vi "Calibration.vi"() -> ()   [LabVIEW 2013]
uses:
  <vilib>/Rock Robotics/WPI/Joystick/WPI_JoystickGetSetRefNum.vi
  Globals/Useful Values.vi
  Globals/Homes.vi
  <vilib>/Utility/file.llb/Write To Spreadsheet File (DBL).vi
panel:
  out "Winch Home":dbl=0.95
  out "Intake Home":dbl=0.1
  out "Arm Home":dbl=0.4
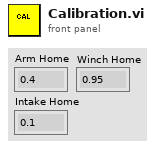
[diagram p1: front panel]
types:
  T1 = typedef "WPI_AnalogChannelDevRef.ctl" = cluster{"DevStatus":errorcluster, "Analog Module":T2, "Analog Channel":T3}
  T2 = typedef "FPGA_TypedefAnalogModule.ctl" = enum16{"Analog Module 1", "Analog Module 2"}
  T3 = typedef "FPGA_AIChannel.ctl" = enum8{"AI 1", "AI 2", "AI 3", "AI 4", "AI 5", "AI 6", "AI 7", "AI 8", "Invalid"}
  T4 = typedef "WPI_JoystickDevRef.ctl" = cluster{"Device":T5}
  T5 = typedef "WPI_JoystickDeviceEnum.ctl" = enum16{"USB 1", "USB 2", "USB 3", "USB 4", "Kinect 1", "Kinect 2"}
  T6 = typedef "WPI_MotorControlDeviceRef.ctl" = cluster{"DeviceStatus":errorcluster, "Type":enum16{"PWM", "CAN"}, "PWM":cluster{"Digital Module":T7, "PWM Channel":T8, "DeadBand":T9}, "CAN":cluster{"Device Number":u8, "Control Mode":T10, "Semaphore":T11, "Max Vout":dbl}, "Invert":bool, "TransformRef":T12, "InvTransformRef":T12}
  T7 = typedef "FPGA_TypedefDigitalModule.ctl" = enum16{"Digital Module 1", "Digital Module 2"}
  T8 = typedef "FPGA_DIOPWMChannel.ctl" = enum8{"PWM 1", "PWM 2", "PWM 3", "PWM 4", "PWM 5", "PWM 6", "PWM 7", "PWM 8", "PWM 9", "PWM 10", "Invalid"}
  T9 = typedef "WPI_PWMDeadband.ctl" = cluster{"Name":string, "maxPositivePwm":i32, "minPositivePwm":i32, "centerPwm":i32, "maxNegativePwm":i32, "minNegativePwm":i32, "angularRange":u16}
  T10 = typedef "WPI_CANJaguar_ControlMode.ctl" = enum8{"Percent VBus", "Current", "Speed", "Position", "Voltage"}
  T11 = typedef "Semaphore RefNum" = refnum<k1>
  T12 = typedef "WPI_PWMTransform_ConPane.ctl" = refnum<vi>
  T13 = typedef "WPI_JoystickButtonState.ctl" = cluster{"Button 1":bool, "Button 2":bool, "Button 3":bool, "Button 4":bool, "Button 5":bool, "Button 6":bool, "Button 7":bool, "Button 8":bool, "Button 9":bool, "Button 10":bool, "Button 11":bool, "Button 12":bool}
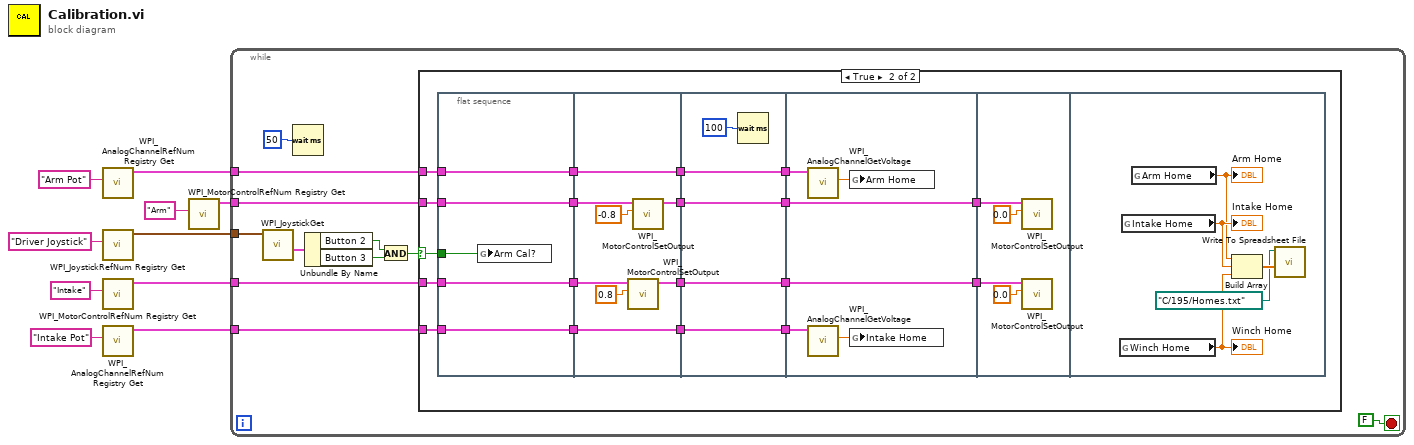
[diagram p0: block diagram]
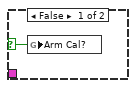
[diagram p2: hidden frame]
diagram:
  n1 = call <vilib>:"WPI_AnalogChannelRefNum Registry Get.vi"("refnum name"="Arm Pot") -> ("AIDeviceRef"=w7:T1)  [unwired: 9 in, 1 out]
  n2 = call <vilib>:"WPI_JoystickRefNum Registry Get.vi"("refnum name"="Driver Joystick") -> ("JoystickDevRef"=w10:T4)  [unwired: 9 in, 1 out]
  n3 = call <vilib>:"WPI_MotorControlRefNum Registry Get.vi"("refnum name"="Intake") -> ("MotorControlDevRef"=w2:T6)  [unwired: 9 in, 1 out]
  n4 = call <vilib>:"WPI_AnalogChannelRefNum Registry Get.vi"("refnum name"="Intake Pot") -> ("AIDeviceRef"=w1:T1)  [unwired: 9 in, 1 out]
  n5 = call <vilib>:"WPI_MotorControlRefNum Registry Get.vi"("refnum name"="Arm") -> ("MotorControlDevRef"=w5:T6)  [unwired: 9 in, 1 out]
  n6 = while {
    tunnel: w10 -> [w20]
    tunnel: w7 -> [w16]
    tunnel: w5 -> [w15]
    tunnel: w2 -> [w12]
    tunnel: w1 -> [w11]
    stop <- FALSE stop-if-true
    n7 = call <vilib>:"WPI_JoystickGet.vi"("JoystickDevRef"=w20) -> ("Buttons"=w19:T13)  [unwired: 4 in, 2 out]
    n8 = Wait (ms)(milliseconds to wait=u32 50) -> ()  [unwired: 1 out]
    n9 = Unbundle By Name(w19) -> ("Button 2"=w18:bool, "Button 3"=w17:bool)
    n10 = And(x=w18, y=w17) -> (x .and. y?=w14:bool)
    n11 = case shown="True" w14 {
      selector: w14 -> [w22 w41]
      tunnel: w16 -> [_ w40]
      tunnel: w15 -> [_ w39]
      tunnel: w12 -> [_ w30]
      tunnel: w11 -> [_ w26]
      frame False {
        n12 = global write "Useful Values.vi" "Arm Cal?"(w22) -> ()
      }
      frame True {
        n13 = flat-sequence {
          tunnel: w41 -> [w46]
          tunnel: [w45] -> w38
          tunnel: w40 -> [w45]
          tunnel: w39 -> [w44]
          tunnel: [w44] -> w37
          tunnel: [w43] -> w31
          tunnel: w30 -> [w43]
          tunnel: [w42] -> w27
          tunnel: w26 -> [w42]
          tunnel: w38 -> [w54]
          tunnel: [w54] -> w35
          tunnel: w37 -> [w52]
          tunnel: [w51] -> w33
          tunnel: w31 -> [w50]
          tunnel: [w48] -> w28
          tunnel: w27 -> [w48]
          tunnel: [w47] -> w25
          tunnel: w35 -> [w59]
          tunnel: [w59] -> w34
          tunnel: w33 -> [w58]
          tunnel: [w58] -> w32
          tunnel: [w56] -> w29
          tunnel: w28 -> [w56]
          tunnel: w25 -> [w55]
          tunnel: [w55] -> w24
          tunnel: w34 -> [w63]
          tunnel: [w65] -> w36
          tunnel: w32 -> [w65]
          tunnel: w29 -> [w62]
          tunnel: w24 -> [w60]
          tunnel: [w60] -> w23
          tunnel: w36 -> [w68]
          tunnel: w23 -> [w66]
          frame #0 {
            n14 = global write "Useful Values.vi" "Arm Cal?"(w46) -> ()
          }
          frame #1 {
            n15 = call <vilib>:"WPI_MotorControlSetOutput.vi"("Output"=0.8, "MotorControlDevRef"=w50) -> ("MotorControlDevRef"=w47:T6)  [unwired: 7 in, 2 out]
            n16 = call <vilib>:"WPI_MotorControlSetOutput.vi"("Output"=-0.8, "MotorControlDevRef"=w52) -> ("MotorControlDevRef"=w51:T6)  [unwired: 7 in, 2 out]
          }
          frame #2 {
            n17 = Wait (ms)(milliseconds to wait=u32 100) -> ()  [unwired: 1 out]
          }
          frame #3 {
            n18 = call <vilib>:"WPI_AnalogChannelGetVoltage.vi"("AIDeviceRef"=w63) -> ("Voltage"=w64:dbl)  [unwired: 8 in, 2 out]
            n19 = call <vilib>:"WPI_AnalogChannelGetVoltage.vi"("AIDeviceRef"=w62) -> ("Voltage"=w61:dbl)  [unwired: 8 in, 2 out]
            n20 = global write "Homes.vi" "Arm Home"(w64) -> ()
            n21 = global write "Homes.vi" "Intake Home"(w61) -> ()
          }
          frame #4 {
            n22 = call <vilib>:"WPI_MotorControlSetOutput.vi"("Output"=0.0, "MotorControlDevRef"=w68) -> ()  [unwired: 7 in, 3 out]
            n23 = call <vilib>:"WPI_MotorControlSetOutput.vi"("Output"=0.0, "MotorControlDevRef"=w66) -> ()  [unwired: 7 in, 3 out]
          }
          frame #5 {
            n24 = global read "Homes.vi" "Winch Home"() -> (w70:dbl)
            "Winch Home" <- w70
            n25 = global read "Homes.vi" "Intake Home"() -> (w74:dbl)
            "Intake Home" <- w74
            n26 = global read "Homes.vi" "Arm Home"() -> (w72:dbl)
            "Arm Home" <- w72
            n27 = Build Array(w72, w74, w70) -> (w73:dbl[])
            n28 = call-poly <vilib>:"Write To Spreadsheet File.vi"("1D data"=w73, "file path (dialog if empty)"=path "C:/195/Homes.txt") -> ()  [unwired: 6 in, 1 out]
          }
        }
      }
    }
  }
